vi "get available list item.vi"(8 "error in (no error)":errorcluster, 11 "available tags list":refnum<vi>) -> (0 "error out":errorcluster, 2 "data type":T1, 3 "element name":string)   [LabVIEW 2014, in "Shared Memory editor node.lvclass"]
uses:
  Shared Memory editor node.lvclass
  <vilib>/NI/Tag Bus/tag/Data Type.ctl
  <vilib>/NI/Tag Bus/tag/tag descriptor.lvclass
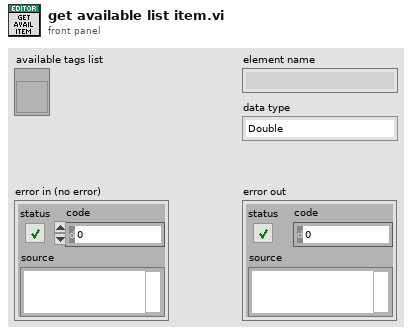
[diagram p1: front panel]
types:
  T1 = typedef "tag bus.lvlib/tag descriptor.lvclass/Data Type.ctl" = enum16{"Double", "Single", "I64", "I32", "I16", "I8", "U64", "U32", "U16", "U8", "Boolean", "String", "Array of Double", "Array of Single", "Array of I64", "Array of I32", "Array of I16", "Array of I8", "Array of U64", "Array of U32", "Array of U16", "Array of U8", "Array of Boolean", "Array of String"}
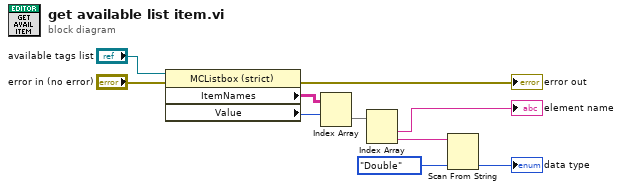
[diagram p0: block diagram]
diagram:
  n1 = property class="MCListbox (strict)"(reference="available tags list", error in="error in (no error)") -> (error out=→"error out":errorcluster, "ItemNames"=w10:string[][], "Value"=w9:i32)  [unwired: 1 out]
  n2 = Index Array(array=w10, index (row)=w9) -> (element=w6:string[])  [unwired: 1 in]
  n3 = Index Array(array=w6) -> (element #1=→"element name":string, element #2=w8:string)  [unwired: 2 in]
  n4 = Scan From String(input string=w8, default 1=Data_Type."Double" ("data type")) -> (output 1=→"data type":T1)  [unwired: 3 in, 3 out]
